vi "SQLite Delete Template.vi"(8 "error in":errorcluster, 10 "PK":cluster{}, 11 "SQLite Connection in":refnum<class "Connection.lvclass">) -> (0 "error out":errorcluster, 3 "SQLite Connection out":refnum<class "Connection.lvclass">)   [LabVIEW 2021]
uses:
  <vilib>/drjdpowell/SQLite Library/SQL Connection/Connection.lvclass
  <vilib>/drjdpowell/SQLite Library/SQL Statement/SQL Statement.lvclass
  edt.lib/sqlite.lib/EDT SQLite+.lvlib
  <vilib>/drjdpowell/SQLite Library/Transaction Helpers/Transaction.lvlib
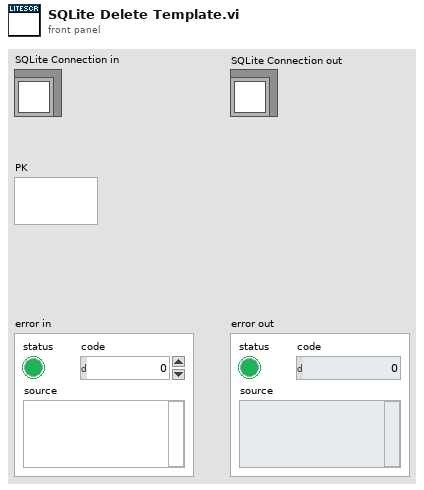
[diagram p1: front panel]
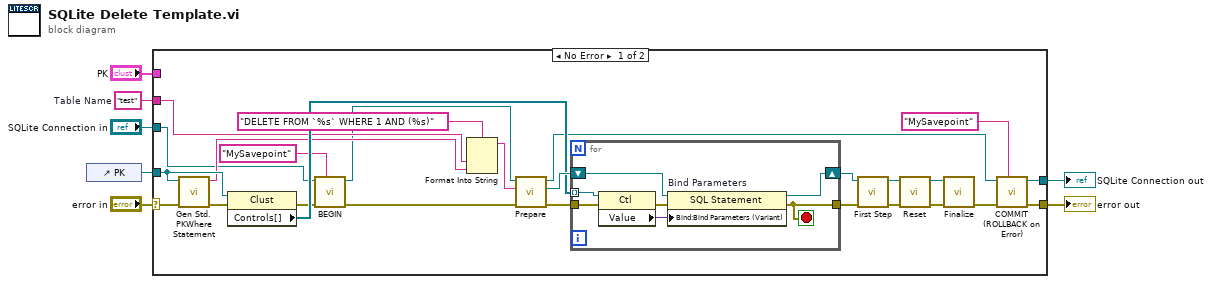
[diagram p0: block diagram]
diagram:
  w2 = "test"  # Table Name
  n1 = control-ref of="PK"() -> (w1:refnum<vi>)
  n2 = case shown="No Error" "error in" {
    selector: "error in" -> [w31 w42]
    tunnel: [w14 w42] -> w6
    tunnel: "PK" -> [_ _]
    tunnel: "SQLite Connection in" -> [w23 w41]
    tunnel: [w15 w41] -> w3
    tunnel: w2 -> [w27 _]
    tunnel: w1 -> [w30 _]
    frame No Error {
      n3 = call "Gen Std.PKWhere Statement.vi"("error in"=w31, "Cluster in"=w30) -> ("error out"=w28:errorcluster, "delimited string"=w26:string)  [unwired: 8 in]
      n4 = property on="Property Node" class="Clust"(reference=w30, error in=w28) -> (error out=w20:errorcluster, "Controls[]"=w29:refnum<vi>[])  [unwired: 1 out]
      n5 = call <vilib>:"BEGIN.vi"("Savepoint name"="MySavepoint", "error in (no error)"=w20, "SQLite Connection in"=w23) -> ("error out"=w21:errorcluster, "SQLite Connection"=w22:refnum<class "Connection.lvclass">)  [unwired: 7 in]
      n6 = Format Into String(format string="DELETE FROM `%s` WHERE 1 AND (%s)" ("SELECT  statement"), w27, w26) -> (resulting string=w25:string)  [unwired: 2 in, 1 out]
      n7 = call <vilib>:"Prepare.vi"("error in (no error)"=w21, "SQL"=w25, "SQLite Connection in"=w22) -> ("error out"=w33:errorcluster, "SQL Statement"=w32:refnum<class "SQL Statement.lvclass">, "SQLite Connection"=w17:refnum<class "Connection.lvclass">)  [unwired: 4 in, 2 out]
      n8 = for {
        shift-right: [w40] -> w11
        shift-left: w32 -> [w39]
        tunnel: w29 -> [w38] mode=indexing
        tunnel: w33 -> [w36]
        tunnel: [w34] -> w10
        stop <- w34 stop-if-true
        n9 = property class="Ctl"(reference=w38, error in=w36) -> (error out=w35:errorcluster, "Value"=w37:variant)  [unwired: 1 out]
        n10 = property on="Bind Parameters" class="SQL Statement"(reference=w39, error in=w35, "Bind:Bind Parameters (Variant)"=w37) -> (reference out=w40:refnum<class "SQL Statement.lvclass">, error out=w34:errorcluster)
      }
      n11 = call <vilib>:"First Step.vi"("error in (no error)"=w10, "SQL Statement in"=w11) -> ("error out"=w13:errorcluster, "SQL Statement"=w12:refnum<class "SQL Statement.lvclass">)  [unwired: 7 in, 1 out]
      n12 = call <vilib>:"Reset.vi"("error in (no error)"=w13, "SQL Statement in"=w12) -> ("error out"=w8:errorcluster, "SQL Statement"=w9:refnum<class "SQL Statement.lvclass">)  [unwired: 8 in]
      n13 = call <vilib>:"Finalize.vi"("error in (no error)"=w8, "SQL Statement in"=w9) -> ("error out"=w18:errorcluster)  [unwired: 9 in]
      n14 = call <vilib>:"COMMIT (ROLLBACK on Error).vi"("Savepoint name"="MySavepoint", "error in (no error)"=w18, "SQLite Connection in"=w17) -> ("error out"=w14:errorcluster, "SQLite Connection"=w15:refnum<class "Connection.lvclass">)  [unwired: 7 in]
    }
    frame Error {
    }
  }
  "error out" <- w6
  "SQLite Connection out" <- w3
